vi "String - Mouse Down.vi"(8 "error in (no error)":errorcluster, 11 "Loop data in":T1={"Config"={"List"=[], "max rows"=8, "Listbox placement"=enum."None", "String Color Options"={"Use? (F)"=FALSE, "Color - Valid"=0, "Color - Invalid"=0, "Allow blank?"=FALSE}}, "Refs"={"String"=refnum, "Listbox"=refnum}, "State"={"LB active?"=FALSE}}) -> (0 "error out":errorcluster, 3 "Loop data out":T1={"Config"={"List"=[], "max rows"=8, "Listbox placement"=enum."None", "String Color Options"={"Use? (F)"=FALSE, "Color - Valid"=0, "Color - Invalid"=0, "Allow blank?"=FALSE}}, "Refs"={"String"=refnum, "Listbox"=refnum}, "State"={"LB active?"=FALSE}})   [LabVIEW 2021, in "Autocomplete Textbox.lvlib"]
uses:
  Autocomplete Textbox.lvlib
  Loop Data.ctl
  Inputs.ctl
  Classes/Handle/Listbox placement.ctl
  Color String Options.ctl
  Refs.ctl
  State data.ctl
  Classes/Handle/Handle.lvclass
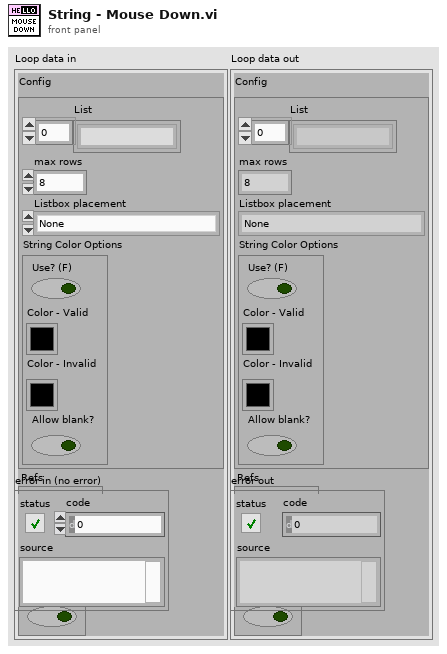
[diagram p1: front panel]
types:
  T1 = typedef "Autocomplete Textbox.lvlib/Loop Data.ctl" = cluster{"Config":T2, "Refs":T5, "State":T6}
  T2 = typedef "Autocomplete Textbox.lvlib/Inputs.ctl" = cluster{"List":string[], "max rows":i32, "Listbox placement":T3, "String Color Options":T4}
  T3 = typedef "Autocomplete Textbox.lvlib/Handle.lvclass/Listbox placement.ctl" = enum16{"None", "Under String", "Fit to Pane"}
  T4 = typedef "Autocomplete Textbox.lvlib/Color String Options.ctl" = cluster{"Use? (F)":bool, "Color - Valid":u32, "Color - Invalid":u32, "Allow blank?":bool}
  T5 = typedef "Autocomplete Textbox.lvlib/Refs.ctl" = cluster{"String":refnum<vi>, "Listbox":refnum<vi>}
  T6 = typedef "Autocomplete Textbox.lvlib/State data.ctl" = cluster{"LB active?":bool}
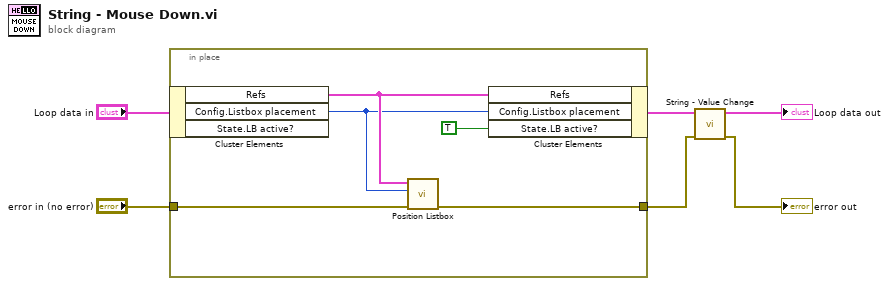
[diagram p0: block diagram]
diagram:
  n1 = in-place {
    in-place-border: "error in (no error)" -> [w10]
    in-place-border: [w9] -> w2
    n2 = in-place-cluster #1("Loop data in") -> ("Refs"=w11:T5, "Config.Listbox placement"=w7:T3)  [unwired: 1 out]
    n3 = call "Position Listbox.vi"("error in (no error)"=w10, "Listbox placement"=w7, "Refs"=w11) -> ("error out"=w9:errorcluster)  [unwired: 8 in]
    n4 = in-place-cluster #1("Refs"=w11, "Config.Listbox placement"=w7, "State.LB active?"=TRUE) -> (w4:T1)
  }
  n5 = call "String - Value Change.vi"("error in (no error)"=w2, "Loop data in"=w4) -> ("error out"=→"error out":errorcluster, "Loop data out"=→"Loop data out":T1)  [unwired: 8 in]
